vi "LSX Get Swap ZA.vi"(8 "error in (no error)":errorcluster, 10 "pbSwapZA":i32, 11 "lLSID":i32) -> (0 "error out":errorcluster, 2 "pbSwapZA out":i32, 3 "function return":i32)   [LabVIEW 2016, in "Tango_DLL.lvlib"]
doc: "TANGOAPI int TANGOCALL LSX_GetSwapZA (int lLSID, BOOL *pbSwapZA);"
uses:
  Tango_DLL.lvlib
  2017/Microscope Control/Device Library/Stages/Marzhauser/SCAN IM 120 x 80/Tango DLL VIs/Tango_DLL.dll
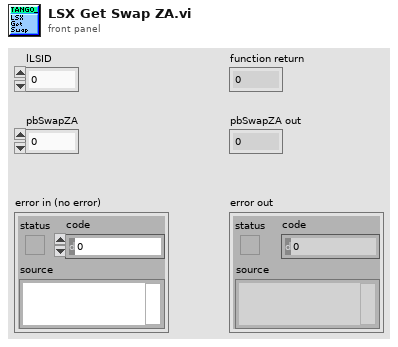
[diagram p1: front panel]
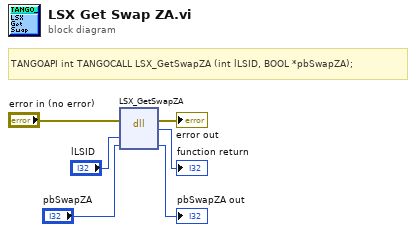
[diagram p0: block diagram]
diagram:
  # "TANGOAPI int TANGOCALL LSX_GetSwapZA (int lLSID, BOOL *pbSwapZA);"
  n1 = dll-call lib="C:/Users/4PiSMS/Documents/Microscope Control/2017/Microscope Control/Device Library/Stages/Marzhauser/SCAN IM 120 x 80/Tango DLL VIs/Tango_DLL.*" fn="LSX_GetSwapZA"(error in="error in (no error)", "lLSID"="lLSID", "pbSwapZA"="pbSwapZA") -> (error out=→"error out":errorcluster, →"function return":i32, "pbSwapZA"=→"pbSwapZA out":i32)  [unwired: 3 in, 1 out]
